vi "fpga 1.vi"() -> ()   [LabVIEW 2015]
uses:
  <vilib>/LabVIEW Targets/FPGA/RIO/nicrio_985x_controls.llb/CAN_IO_Frame Cluster.ctl
  <vilib>/LabVIEW Targets/FPGA/RIO/nicrio_985x_controls.llb/CAN_IO_Frame Type.ctl
  <vilib>/rvi/Emulation/niFpgaGetClockAttributes.vi
  <vilib>/rvi/Emulation/niFpgaSctlEmulationGetInTimedLoop.vi
  <vilib>/rvi/Emulation/niFpgaEmulationReportErrorSimple.vi
  <vilib>/rvi/eio/common/nirviEmuTemplateMethod_errors.vi
  <vilib>/rvi/Emulation/niFpgaCriticalErrorInLSC.vi
  <vilib>/rvi/interface/RandomDataEmulation/niFpgaRandomDataHandleErrors.vi
  <vilib>/rvi/Emulation/niFpgaProcessEmulError.vi
  <vilib>/eio/EIONode/EIONode.xnode
  <vilib>/eio/EIOMethodNode/EIOMethodNode.xnode
  <vilib>/rvi/DataTransferAndStorage/Container/XNode/niFpgaContainer.xnode
  <vilib>/rvi/interface/RandomDataEmulation/nirviRandomDataFpgaReadWriteTemplate.vi
panel:
  in  "Mod1/DIO3":bool
  in  "Mod3/AO3":fxp<+/-,20,5>
  in  "Mod3/AO2":fxp<+/-,20,5>
  in  "Mod3/AO1":fxp<+/-,20,5>
  in  "Mod3/AO0":fxp<+/-,20,5>
  out "CAN1":u8[](array[numeric])
  out "CAN0":u8[](array[numeric])
  in  "Mod2/CAN0 input":T1={"timestamp high"=0, "timestamp low"=0, "identifier"=0, "type"=enum."Data Frame", "info A"=0, "info B"=0, "data length"=0, "data"=[0, 0, 0, 0, 0, 0, 0, 0]} {"identifier" format="%x"; "timestamp high" format="%08x"; "timestamp low" format="%08x"; "data" format="%.0x"}
  in  "send can 0":bool
  in  "send can 1":bool
  in  "Mod2/CAN1 input":T1={"timestamp high"=0, "timestamp low"=0, "identifier"=0, "type"=enum."Data Frame", "info A"=0, "info B"=0, "data length"=0, "data"=[0, 0, 0, 0, 0, 0, 0, 0]} {"identifier" format="%x"; "timestamp high" format="%08x"; "timestamp low" format="%08x"; "data" format="%.0x"}
  out "PWM Read":u16
  out "Mod2/CAN1":T1={"timestamp high"=0, "timestamp low"=0, "identifier"=0, "type"=enum."Data Frame", "info A"=0, "info B"=0, "data length"=0, "data"=[0, 0, 0, 0, 0, 0, 0, 0]} {"identifier" format="%x"; "timestamp high" format="%08x"; "timestamp low" format="%08x"; "data" format="%.0x"}
  out "Mod2/CAN0":T1={"timestamp high"=0, "timestamp low"=0, "identifier"=0, "type"=enum."Data Frame", "info A"=0, "info B"=0, "data length"=0, "data"=[0, 0, 0, 0, 0, 0, 0, 0]} {"identifier" format="%x"; "timestamp high" format="%08x"; "timestamp low" format="%08x"; "data" format="%.0x"}
  out "tmp out":bool
  out "Run":bool
  out "Auto":bool
  in  "Solenoid":bool
  in  "PWM Gas":u16
  in  "PWM Brake":u16
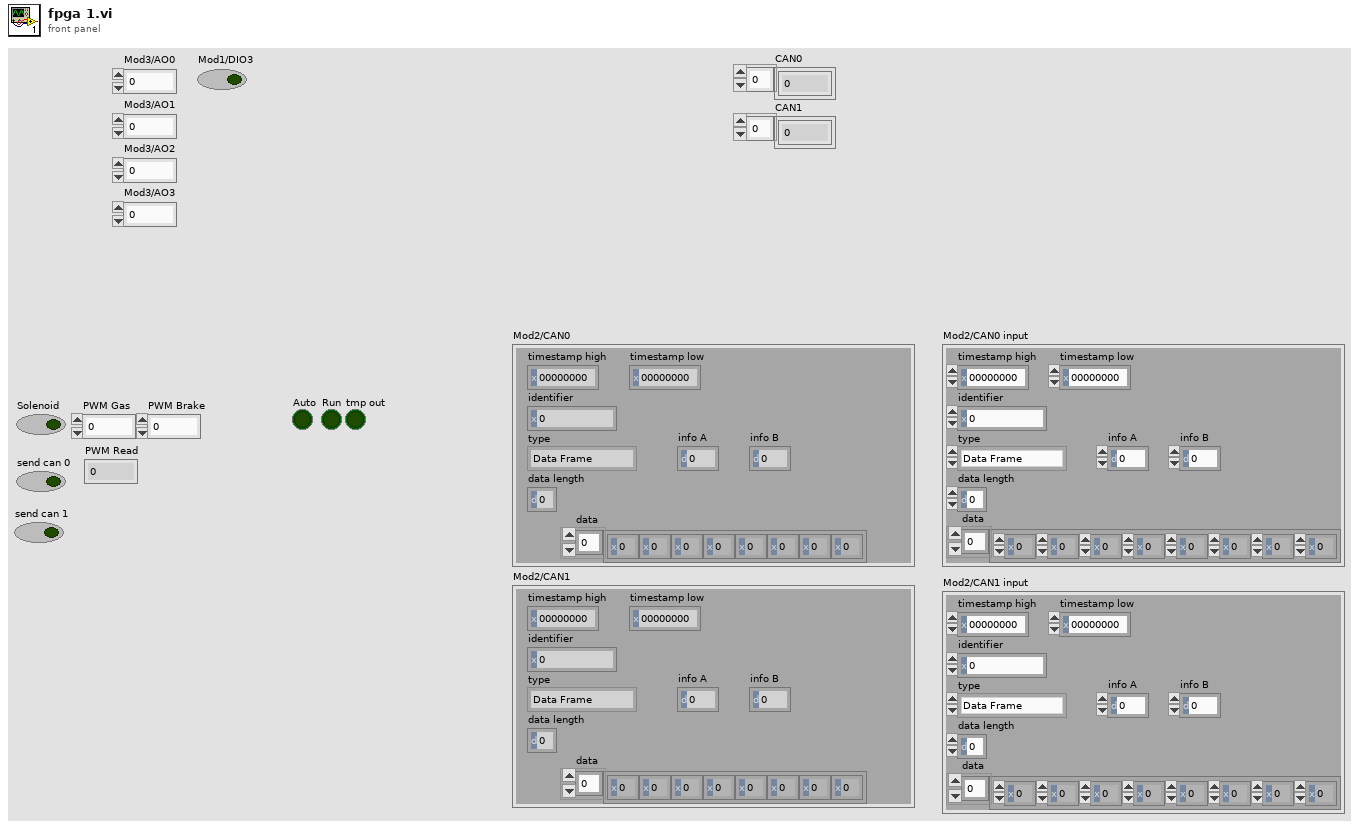
[diagram p1: front panel]
types:
  T1 = typedef "CAN_IO_Frame Cluster.ctl" = cluster{"timestamp high":u32, "timestamp low":u32, "identifier":u32, "type":T2, "info A":u8, "info B":u8, "data length":u8, "data":u8[]}
  T2 = typedef "CAN_IO_Frame Type.ctl" = enum8{"Data Frame", "Remote Frame", "(reserved)", "(reserved) ", "(reserved)  ", "(reserved)   ", "Bus Error", "Transceiver Fault"}
  T3 = cluster{"data[0]":u8, "data[1]":u8, "data[2]":u8, "data[3]":u8, "data[4]":u8, "data[5]":u8, "data[6]":u8, "data[7]":u8}
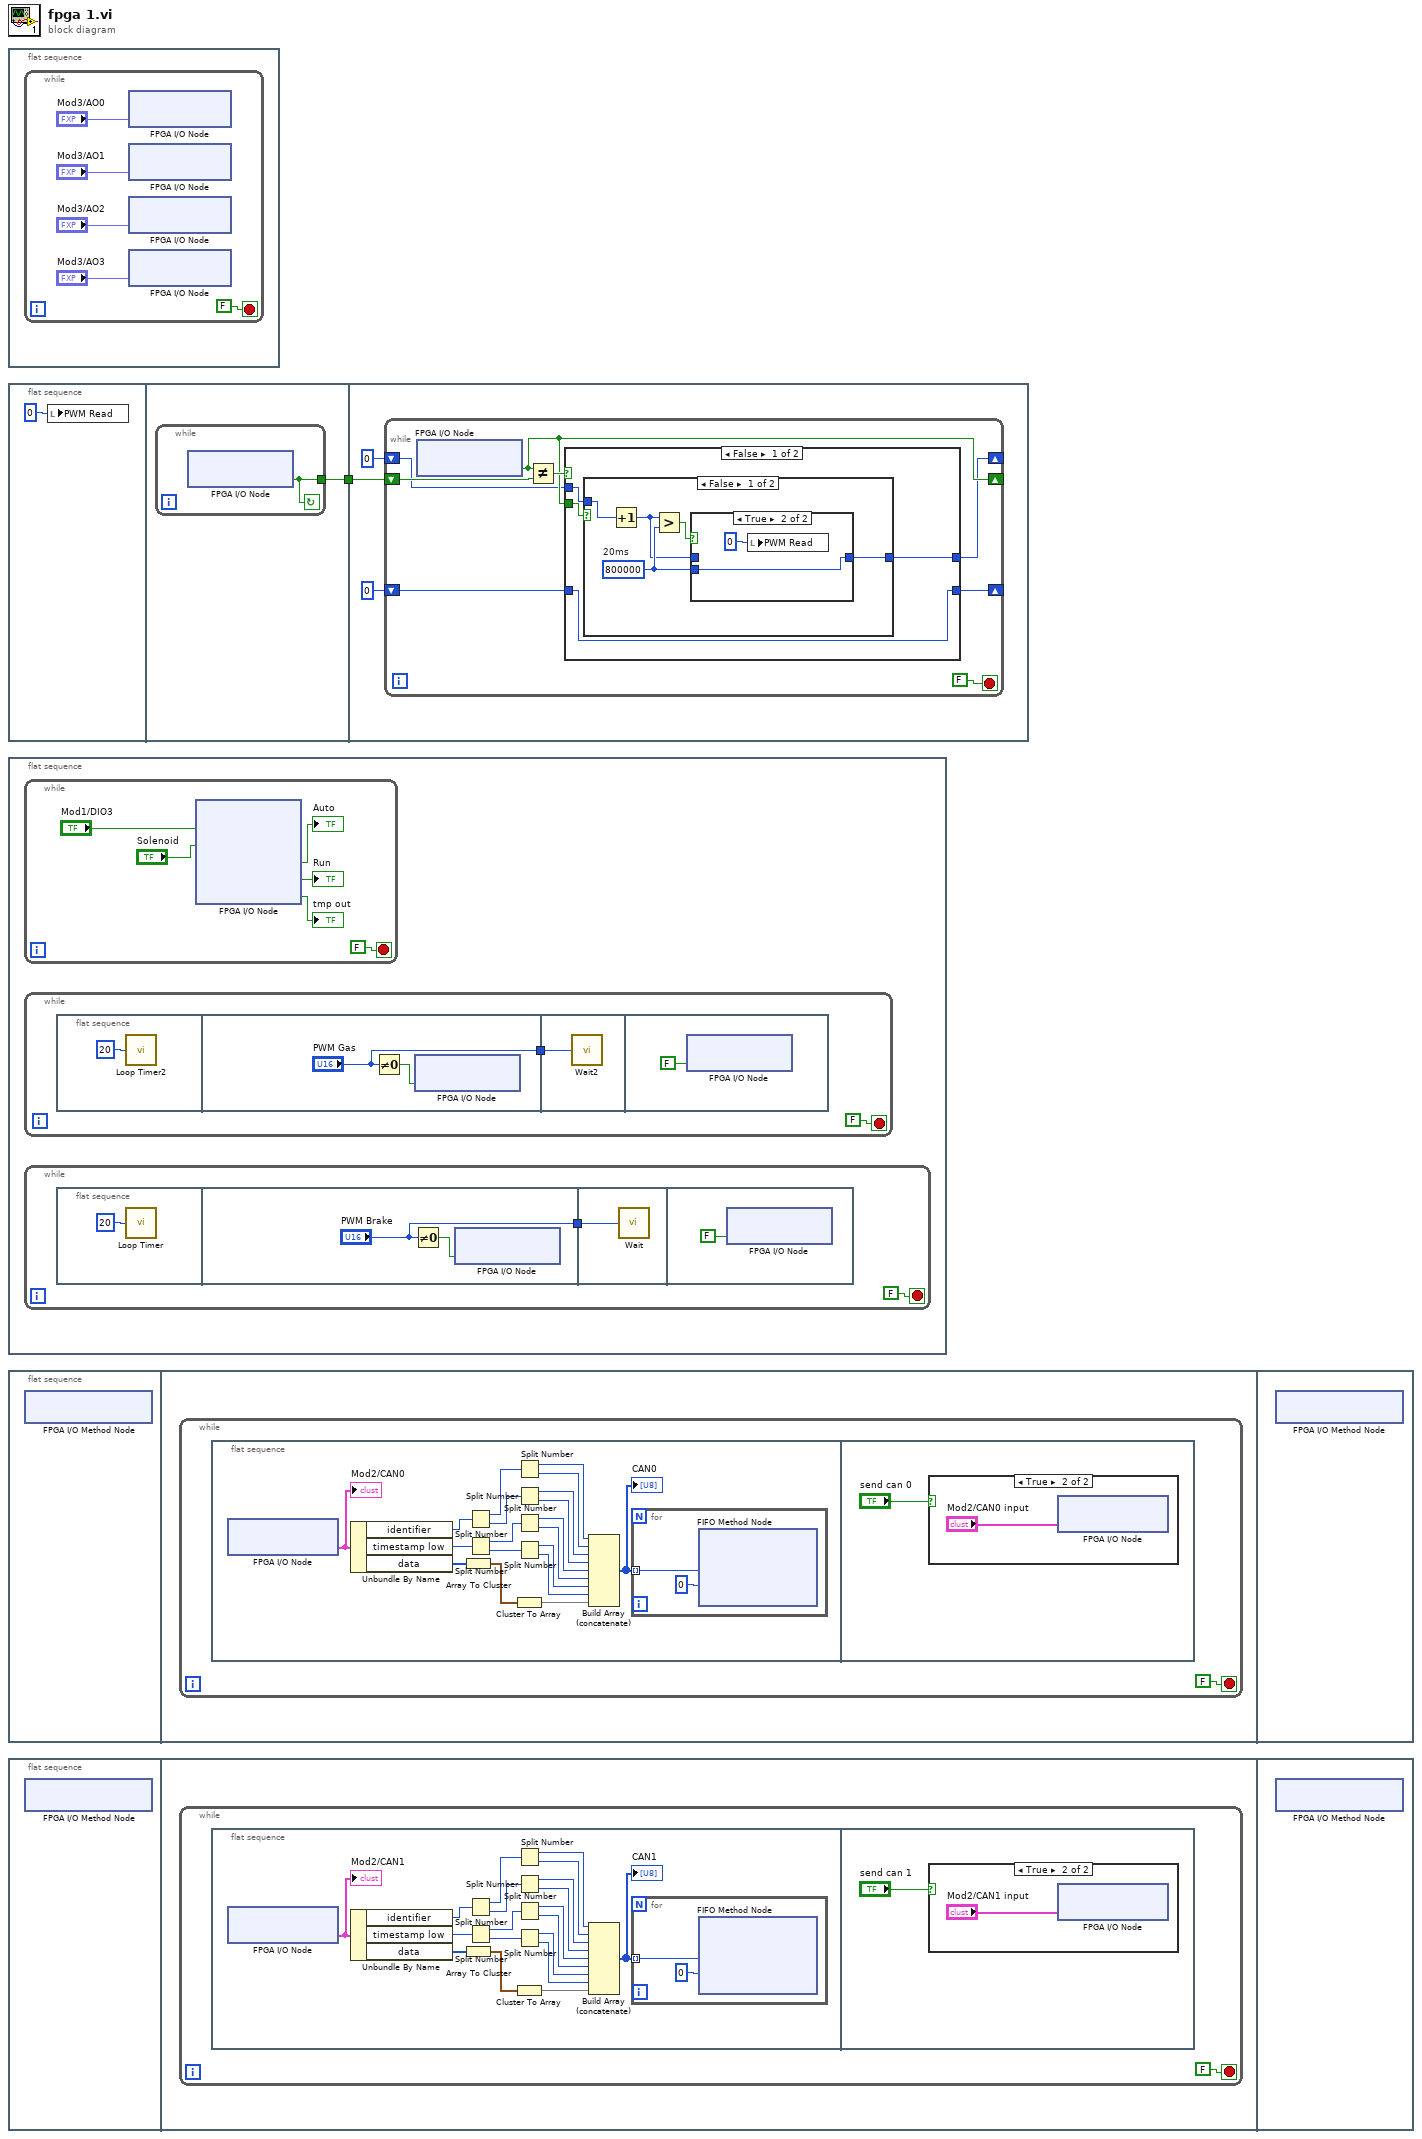
[diagram p0: block diagram]
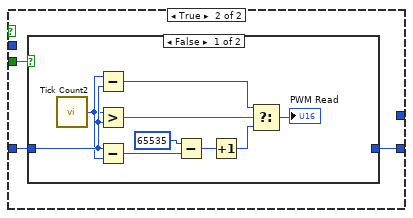
[diagram p4: hidden frame]
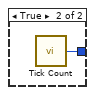
[diagram p5: hidden frame]
diagram:
  n1 = flat-sequence {
    frame #0 {
      n2 = while {
        stop <- FALSE stop-if-true
        n3 = xnode "FPGA I/O Node"("Mod3/AO0"="Mod3/AO0") -> ()  [unwired: 1 in, 1 out]
        n4 = xnode "FPGA I/O Node"("Mod3/AO1"="Mod3/AO1") -> ()  [unwired: 1 in, 1 out]
        n5 = xnode "FPGA I/O Node"("Mod3/AO2"="Mod3/AO2") -> ()  [unwired: 1 in, 1 out]
        n6 = xnode "FPGA I/O Node"("Mod3/AO3"="Mod3/AO3") -> ()  [unwired: 1 in, 1 out]
      }
    }
  }
  n7 = flat-sequence {
    tunnel: [w8] -> w1
    tunnel: w1 -> [w12]
    frame #0 {
      n8 = local write "PWM Read"(u16 0 ("PWM Read")) -> ()
    }
    frame #1 {
      n9 = while {
        tunnel: [w9] -> w8
        stop <- w9 continue-if-true
        n10 = xnode "FPGA I/O Node"() -> ("Mod1/DIO7"=w9:bool)  [unwired: 1 in, 1 out]
      }
    }
    frame #2 {
      n11 = while {
        shift-right: [w15] -> _
        shift-left: w12 -> [w16]
        shift-right: [w19] -> _
        shift-left: u16 0 ("Tick Count(uSec)") -> [w17]
        shift-right: [w13] -> _
        shift-left: u32 0 ("Tick Count(mSec)") -> [w14]
        stop <- FALSE stop-if-true
        n12 = xnode "FPGA I/O Node"() -> ("Mod1/DIO7"=w15:bool)  [unwired: 1 in, 1 out]
        n13 = Not Equal?(x=w15, y=w16) -> (x != y?=w18:bool)
        n14 = case shown="False" w18 {
          tunnel: w15 -> [w23 w35]
          tunnel: [w24 w34] -> w19
          tunnel: w17 -> [w24 w33]
          tunnel: w14 -> [w22 _]
          tunnel: [w21 _] -> w13
          frame False {
            n15 = case shown="False" w23 {
              tunnel: w22 -> [w29 _]
              tunnel: [w27 _] -> w21
              frame False {
                w26 = u32 800000  # 20ms
                n16 = Increment(x=w29) -> (x+1=w25:u32)
                n17 = Greater?(x=w25, y=w26) -> (0:w28:bool)
                n18 = case shown="True" w28 {
                  tunnel: [w30 w31] -> w27
                  tunnel: w26 -> [_ w31]
                  tunnel: w25 -> [w30 _]
                  frame False {
                  }
                  frame True {
                    n19 = local write "PWM Read"(u16 0 ("PWM Read")) -> ()
                  }
                }
              }
              frame True {
              }
            }
          }
          frame True {
            n20 = case shown="False" w35 {
              tunnel: [_ w45] -> w34
              tunnel: w33 -> [w42 _]
              frame False {
                n21 = call "Tick Count2"() -> ("Tick Count(uSec)"=w41:u16)
                n22 = Subtract(x=w41, y=w42) -> (x-y=w43:u16)
                n23 = Greater?(x=w41, y=w42) -> (0:w44:bool)
                n24 = Subtract(x=w42, y=w41) -> (x-y=w40:u16)
                n25 = Subtract(x=u16 65535, y=w40) -> (x-y=w38:u16)
                n26 = Increment(x=w38) -> (x+1=w37:u16)
                n27 = Select(t=w43, s=w44, f=w37) -> (s? t:f=→"PWM Read":u16)
              }
              frame True {
                n28 = call "Tick Count"() -> ("Tick Count(uSec)"=w45:u16)
              }
            }
          }
        }
      }
    }
  }
  n29 = flat-sequence {
    frame #0 {
      n30 = while {
        stop <- FALSE stop-if-true
        n31 = xnode "FPGA I/O Node"("Mod1/DIO3"="Mod1/DIO3", "Mod1/DIO0"="Solenoid") -> ("Mod1/DIO4"=→"Auto":bool, "Mod1/DIO5"=→"Run":bool, "Mod1/DIO6"=→"tmp out":bool)  [unwired: 5 in, 5 out]
      }
      n32 = while {
        stop <- FALSE stop-if-true
        n33 = flat-sequence {
          tunnel: ["PWM Gas"] -> w52
          tunnel: w52 -> [w57]
          frame #0 {
            n34 = call "Loop Timer2"("Count(mSec)"=u16 20) -> ()  [unwired: 1 out]
          }
          frame #1 {
            n35 = Not Equal To 0?(x="PWM Gas") -> (x != 0?=w56:bool)
            n36 = xnode "FPGA I/O Node"("Mod1/DIO1"=w56) -> ()  [unwired: 1 in, 1 out]
          }
          frame #2 {
            n37 = call "Wait2"("Count(uSec)"=w57) -> ()  [unwired: 1 out]
          }
          frame #3 {
            n38 = xnode "FPGA I/O Node"("Mod1/DIO1"=FALSE ("Mod1/DIO0")) -> ()  [unwired: 1 in, 1 out]
          }
        }
      }
      n39 = while {
        stop <- FALSE stop-if-true
        n40 = flat-sequence {
          tunnel: ["PWM Brake"] -> w59
          tunnel: w59 -> [w64]
          frame #0 {
            n41 = call "Loop Timer"("Count(mSec)"=u16 20) -> ()  [unwired: 1 out]
          }
          frame #1 {
            n42 = Not Equal To 0?(x="PWM Brake") -> (x != 0?=w63:bool)
            n43 = xnode "FPGA I/O Node"("Mod1/DIO2"=w63) -> ()  [unwired: 1 in, 1 out]
          }
          frame #2 {
            n44 = call "Wait"("Count(uSec)"=w64) -> ()  [unwired: 1 out]
          }
          frame #3 {
            n45 = xnode "FPGA I/O Node"("Mod1/DIO2"=FALSE ("Mod1/DIO0")) -> ()  [unwired: 1 in, 1 out]
          }
        }
      }
    }
  }
  n46 = flat-sequence {
    frame #0 {
      n47 = xnode "FPGA I/O Method Node"() -> ()  [unwired: 1 in, 1 out]
    }
    frame #1 {
      n48 = while {
        stop <- FALSE stop-if-true
        n49 = flat-sequence {
          frame #0 {
            n50 = xnode "FPGA I/O Node"() -> ("Mod2/CAN0"=w85:T1)  [unwired: 1 in, 1 out]
            "Mod2/CAN0" <- w85
            n51 = Unbundle By Name(w85) -> ("identifier"=w69:u32, "timestamp low"=w68:u32, "data"=w67:u8[])
            n52 = Array To Cluster(array=w67) -> (cluster=w72:T3)
            n53 = Split Number(x=w69) -> (hi(x)=w80:u16, lo(x)=w79:u16)
            n54 = Split Number(x=w68) -> (hi(x)=w73:u16, lo(x)=w74:u16)
            n55 = Cluster To Array(cluster=w72) -> (array=w71:u8[])
            n56 = Split Number(x=w80) -> (hi(x)=w84:u8, lo(x)=w83:u8)
            n57 = Split Number(x=w79) -> (hi(x)=w82:u8, lo(x)=w81:u8)
            n58 = Split Number(x=w73) -> (hi(x)=w78:u8, lo(x)=w77:u8)
            n59 = Split Number(x=w74) -> (hi(x)=w76:u8, lo(x)=w75:u8)
            n60 = Build Array (concatenate)(w84, w83, w82, w81, w78, w77, w76, w75, w71) -> (w70:u8[])
            "CAN0" <- w70
            n61 = for {
              tunnel: w70 -> [w87] mode=indexing
              n62 = xnode ("FIFO Method Node")("Element"=w87, "Timeout"=0) -> ()  [unwired: 1 in, 2 out]
            }
          }
          frame #1 {
            n63 = case shown="True" "send can 0" {
              frame False {
              }
              frame True {
                n64 = xnode "FPGA I/O Node"("Mod2/CAN0"="Mod2/CAN0 input") -> ()  [unwired: 1 in, 1 out]
              }
            }
          }
        }
      }
    }
    frame #2 {
      n65 = xnode "FPGA I/O Method Node"() -> ()  [unwired: 1 in, 1 out]
    }
  }
  n66 = flat-sequence {
    frame #0 {
      n67 = xnode "FPGA I/O Method Node"() -> ()  [unwired: 1 in, 1 out]
    }
    frame #1 {
      n68 = while {
        stop <- FALSE stop-if-true
        n69 = flat-sequence {
          frame #0 {
            n70 = xnode "FPGA I/O Node"() -> ("Mod2/CAN1"=w109:T1)  [unwired: 1 in, 1 out]
            "Mod2/CAN1" <- w109
            n71 = Unbundle By Name(w109) -> ("identifier"=w95:u32, "timestamp low"=w104:u32, "data"=w105:u8[])
            n72 = Array To Cluster(array=w105) -> (cluster=w107:T3)
            n73 = Split Number(x=w95) -> (hi(x)=w96:u16, lo(x)=w97:u16)
            n74 = Split Number(x=w104) -> (hi(x)=w103:u16, lo(x)=w102:u16)
            n75 = Cluster To Array(cluster=w107) -> (array=w108:u8[])
            n76 = Split Number(x=w96) -> (hi(x)=w91:u8, lo(x)=w92:u8)
            n77 = Split Number(x=w97) -> (hi(x)=w93:u8, lo(x)=w94:u8)
            n78 = Split Number(x=w103) -> (hi(x)=w98:u8, lo(x)=w99:u8)
            n79 = Split Number(x=w102) -> (hi(x)=w100:u8, lo(x)=w101:u8)
            n80 = Build Array (concatenate)(w91, w92, w93, w94, w98, w99, w100, w101, w108) -> (w106:u8[])
            "CAN1" <- w106
            n81 = for {
              tunnel: w106 -> [w111] mode=indexing
              n82 = xnode ("FIFO Method Node")("Element"=w111, "Timeout"=0) -> ()  [unwired: 1 in, 2 out]
            }
          }
          frame #1 {
            n83 = case shown="True" "send can 1" {
              frame False {
              }
              frame True {
                n84 = xnode "FPGA I/O Node"("Mod2/CAN1"="Mod2/CAN1 input") -> ()  [unwired: 1 in, 1 out]
              }
            }
          }
        }
      }
    }
    frame #2 {
      n85 = xnode "FPGA I/O Method Node"() -> ()  [unwired: 1 in, 1 out]
    }
  }
